vi "6.1 Cluster flatten rulers.vi"() -> ()   [LabVIEW 2017]
uses:
  601d0760-d4b8-4795-a453-687868710894.vi
  39620bd7-9c21-4071-a996-c10094c7c5f6.vi
  6aef6293-1b46-43cc-a090-3bd41170cef4.vi
  c2ea3052-9718-4095-9bf2-a156dcd4a46a.vi
  API-String-Arugments-Support/_Support/Data To API String Arguments.vi
  API-String-Arugments-Support/_Support/Convert API String Arguments to Data(variant).vi
panel:
  out "output cluster":T1={"Data 8"={"Name"="abc", "Child"={"Name"="xxx"}, "Bool"=TRUE}, "Reference cluster in Flatten"={"Name"="abc", "Child"={"Name"="ddd"}, "Bool"=FALSE}, "Flattened String"="{Child.Name:xxx;Bool:TRUE}", "Reference cluster in Retrieve"={"Name"="abc", "Child"={"Name"="ddd"}, "Bool"=FALSE}, "Retrieved Data"={"Name"="abc", "Child"={"Name"="xxx"}, "Bool"=TRUE}}
  out "Flatten Without Reference Cluster":T2={"Original Data"={"Name"="abc", "Child"={"Name"="ddd"}, "Bool"=FALSE}, "Default Reference in Flatten"=variant, "Flattened String"="{Name:abc;Child.Name:ddd;Bool:FALSE}", "Reference cluster in Retrieve"={"Name"="abc", "Child"={"Name"="ddd"}, "Bool"=FALSE}, "Retrieved Data"={"Name"="abc", "Child"={"Name"="ddd"}, "Bool"=FALSE}}
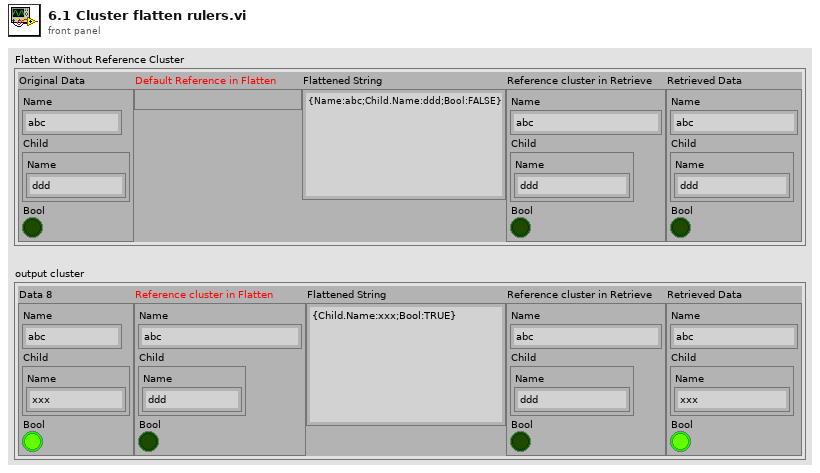
[diagram p1: front panel]
types:
  T1 = cluster{"Data 8":cluster{"Name":string, "Child":cluster{"Name":string}, "Bool":bool}, "Reference cluster in Flatten":cluster{"Name":string, "Child":cluster{"Name":string}, "Bool":bool}, "Flattened String":string, "Reference cluster in Retrieve":cluster{"Name":string, "Child":cluster{"Name":string}, "Bool":bool}, "Retrieved Data":cluster{"Name":string, "Child":cluster{"Name":string}, "Bool":bool}}
  T2 = cluster{"Original Data":cluster{"Name":string, "Child":cluster{"Name":string}, "Bool":bool}, "Default Reference in Flatten":variant, "Flattened String":string, "Reference cluster in Retrieve":cluster{"Name":string, "Child":cluster{"Name":string}, "Bool":bool}, "Retrieved Data":cluster{"Name":string, "Child":cluster{"Name":string}, "Bool":bool}}
  T3 = cluster{"Name":string, "Child":cluster{"Name":string}, "Bool":bool}
  T4 = cluster{"Data 8":cluster{"Name":string, "Child":cluster{"Name":string}, "Bool":bool}, "reference cluster data":variant, "String":string, "Reference cluster data":cluster{"Name":string, "Child":cluster{"Name":string}, "Bool":bool}, "Data":cluster{"Name":string, "Child":cluster{"Name":string}, "Bool":bool}}
  T5 = cluster{"Data 8":cluster{"Name":string, "Child":cluster{"Name":string}, "Bool":bool}, "Reference cluster data":cluster{"Name":string, "Child":cluster{"Name":string}, "Bool":bool}, "String":string, "Reference cluster data":cluster{"Name":string, "Child":cluster{"Name":string}, "Bool":bool}, "Data":cluster{"Name":string, "Child":cluster{"Name":string}, "Bool":bool}}
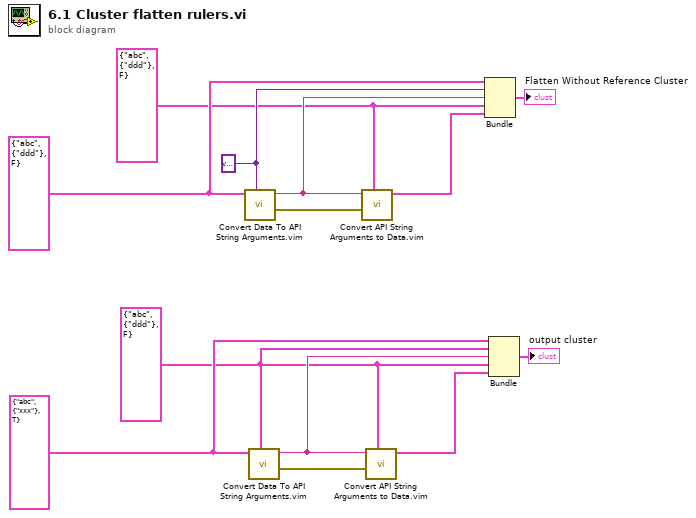
[diagram p0: block diagram]
diagram:
  w2 = T3 {"Name"="abc", "Child"={"Name"="ddd"}, "Bool"=FALSE} ("Reference cluster data")
  w4 = T3 {"Name"="abc", "Child"={"Name"="xxx"}, "Bool"=TRUE} ("Data 8")
  w9 = T3 {"Name"="abc", "Child"={"Name"="ddd"}, "Bool"=FALSE} ("Reference cluster data")
  w11 = variant ("reference cluster data")
  w12 = T3 {"Name"="abc", "Child"={"Name"="ddd"}, "Bool"=FALSE} ("Data 8")
  n1 = call "Convert Data To API String Arguments.vim"("reference cluster data"=w11, "data"=w12) -> ("error out"=w13:errorcluster, "String"=w10:string)  [unwired: 6 in]
  n2 = call "Convert Data To API String Arguments.vim"("reference cluster data"=w2, "data"=w4) -> ("error out"=w3:errorcluster, "String"=w5:string)  [unwired: 6 in]
  n3 = call "Convert API String Arguments to Data.vim"("Type"=w9, "error in (no error)"=w13, "String"=w10) -> ("Data"=w8:T3)  [unwired: 5 in, 1 out]
  n4 = call "Convert API String Arguments to Data.vim"("Type"=w2, "error in (no error)"=w3, "String"=w5) -> ("Data"=w6:T3)  [unwired: 5 in, 1 out]
  n5 = Bundle("Data 8"=w12, "reference cluster data"=w11, "String"=w10, "Reference cluster data"=w9, "Data"=w8) -> (→"Flatten Without Reference Cluster":T4)  [unwired: 1 in]
  n6 = Bundle("Data 8"=w4, "Reference cluster data"=w2, "String"=w5, "Reference cluster data"=w2, "Data"=w6) -> (→"output cluster":T5)  [unwired: 1 in]
